vi "Report port and error.vi"(8 "error in (no error)":errorcluster, 11 "port":u16) -> (0 "error out":errorcluster, 2 "Array":string[](array[string]), 3 "output cluster":cluster{string, "error out":errorcluster})   [LabVIEW 2019]
uses:
  <vilib>/Utility/error.llb/DialogType.ctl
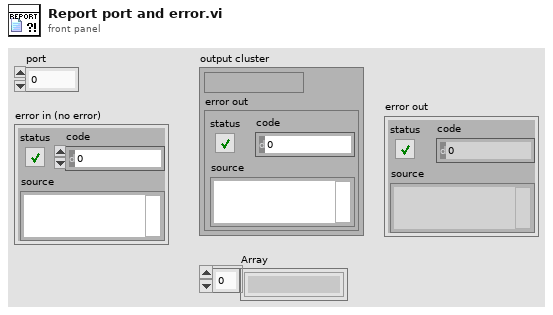
[diagram p1: front panel]
types:
  T1 = typedef "DialogType.ctl" = u16
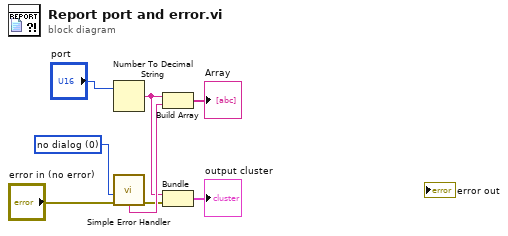
[diagram p0: block diagram]
diagram:
  w4 = T1 0 items=["no dialog", "OK message", "continue or stop message", "OK message + warnings", "continue/stop + warnings"] ("type of dialog (OK msg:1)")
  n1 = Number To Decimal String(number="port") -> (decimal integer string=w5:string)  [unwired: 1 in]
  n2 = call <vilib>:"Simple Error Handler.vi"("type of dialog (OK msg:1)"=w4, "error in (no error)"="error in (no error)") -> ("error out"=w3:errorcluster, "message"=w6:string)  [unwired: 3 in, 3 out]
  n3 = Build Array(w5, w6) -> (→"Array":string[])
  n4 = Bundle(w5, "error out"=w3) -> (→"output cluster":cluster{string, "error out":errorcluster})  [unwired: 1 in]
